vi "test_HM_times_x_preload_N22.vi"() -> ()   [LabVIEW 2017, in "MPC_FXP_FGM_TestCase.lvclass"]
uses:
  MPC_FXP_FGM_TestCase.lvclass
  fpga_VIs/fixed-point/typeDefs/x_vec_type.ctl
  C:/Program Files (x86)/National Instruments/LabVIEW 2017/vi.lib/addons/_JKI Toolkits/VI Tester/TestCase.llb/TestCase.lvclass
  <vilib>/rvi/DesktopExecutionNode/Execution/niFpgaDEN_Execute.vi
  <vilib>/rvi/DesktopExecutionNode/DesktopExecutionNode.xnode
  <userlib>/_VITAC/VITAC.lvlib
panel:
  out "error out":errorcluster
  in  "error in (no error)":errorcluster
  out "MPC_FXP_FGM_TestCase.lvclass 2":refnum<class "MPC_FXP_FGM_TestCase.lvclass">
  in  "MPC_FXP_FGM_TestCase.lvclass":refnum<class "MPC_FXP_FGM_TestCase.lvclass">
  out "all rows":dbl[][](array[numeric])
  out "x_vec":T1=[0.6000000238418579, 0.6000000238418579, -0.5999999940395355, -0.5999999940395355, 0.6000000238418579, 0.6000000238418579, 0.6000000238418579, 0.6000000238418579, -0.5999999940395355, 0.6000000238418579, -0.5999999940395355, -4.0, 0.0, 0.0, 0.0, 0.0, 0.0, 0.0, 0.0, 0.0, 0.0, 0.0, 0.0, 0.0, 0.0]
  out "A*x (expected, fxp)":fxp<+/-,32,3>[](array[numeric])
  out "Ncol":u16
  out "primary_write_addr":u16
  in  "preload_vec":fxp<+/-,32,3>[](array[numeric])=[0.0, 0.0, 0.0, 0.0, 0.0, 0.0, 0.0, 0.0, 0.0, 0.0, 0.0, 0.0, 0.0, 0.0, 0.0, 0.0, 0.0, 0.0, 0.0, 0.0, 0.0, 0.0]
  out "preload_addr":u16
  out "StartIndex":u16
  out "primary result (A*x)":fxp<+/-,32,2>[](array[numeric])
  out "preload result":fxp<+/-,32,2>[](array[numeric])
  in  "SLMAX":fxp<+/-,18,5>=10.0
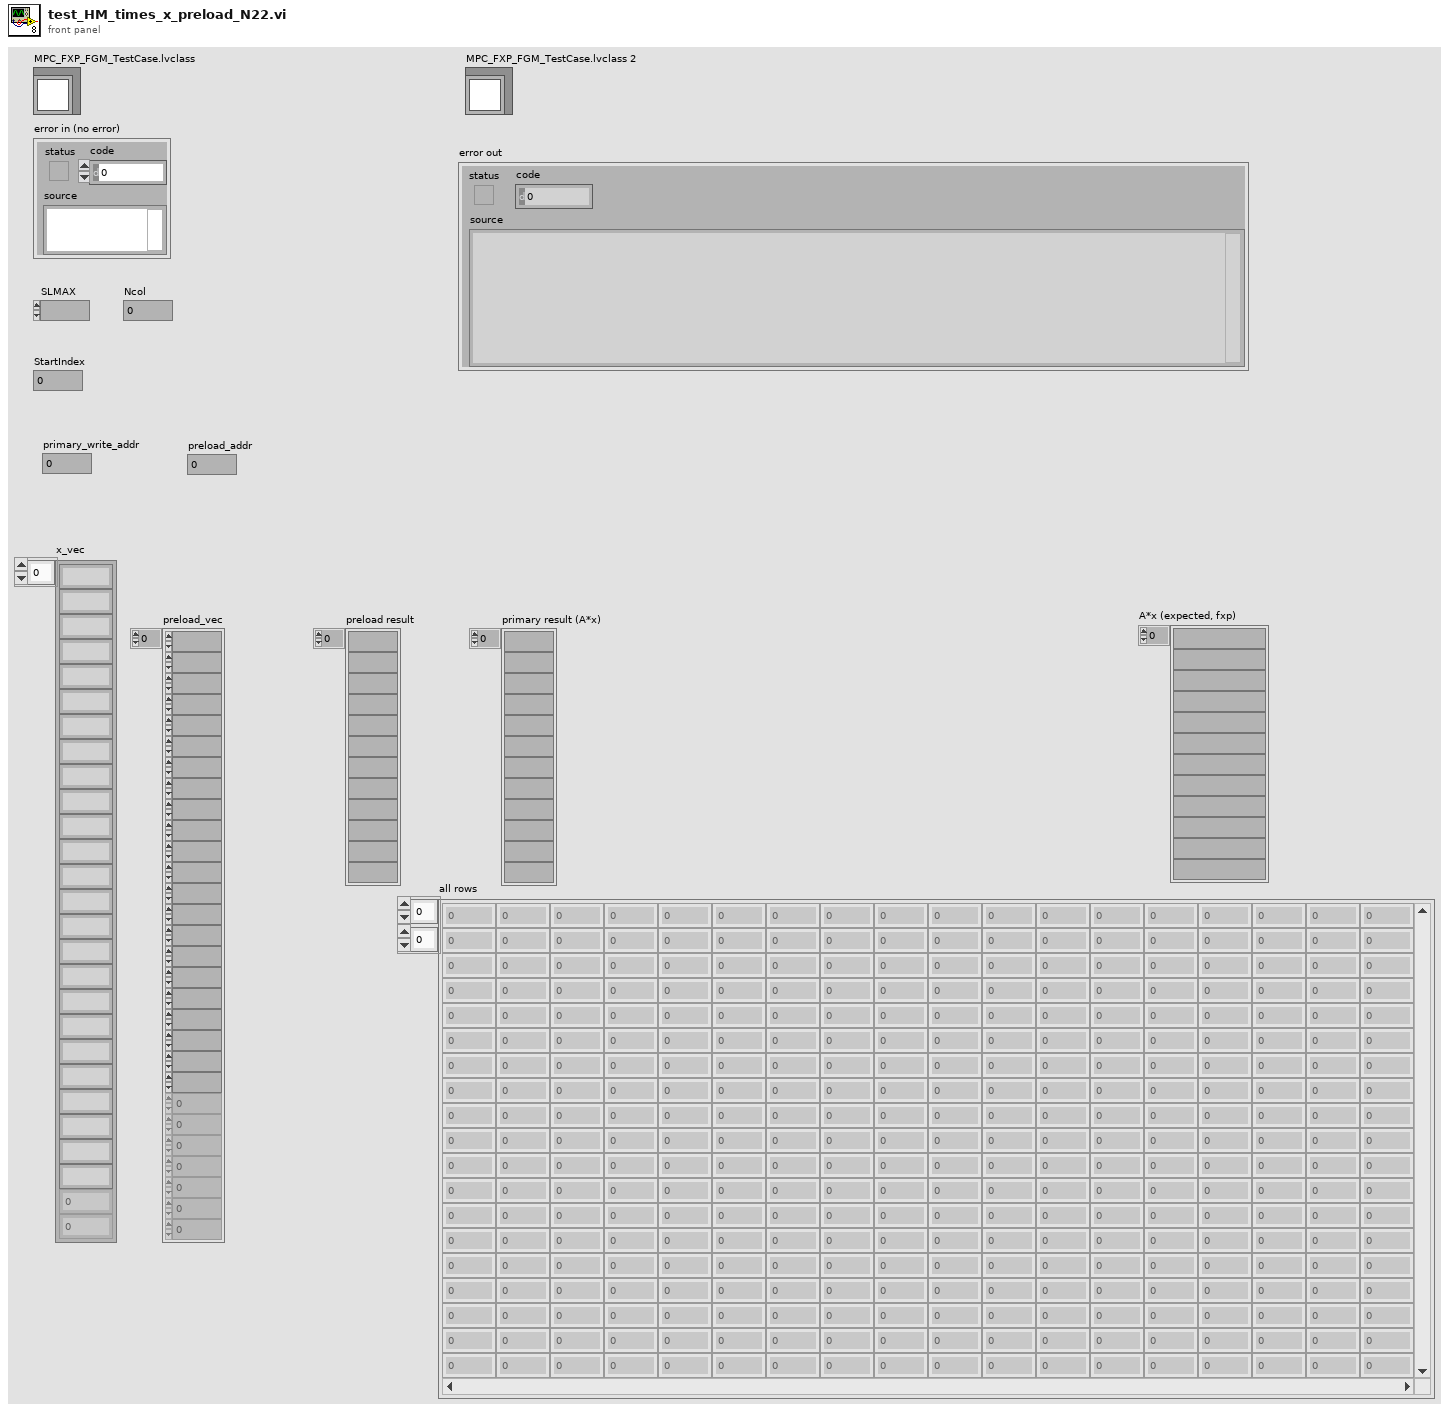
[diagram p1: front panel]
types:
  T1 = typedef "x_vec_type.ctl" = fxp<+/-,32,6>[]
  T2 = typedef "fgm_result_test_data.ctl" = cluster{"z_i_sequence":dbl[][], "y_i_sequence":dbl[][], "X_states":dbl[][]}
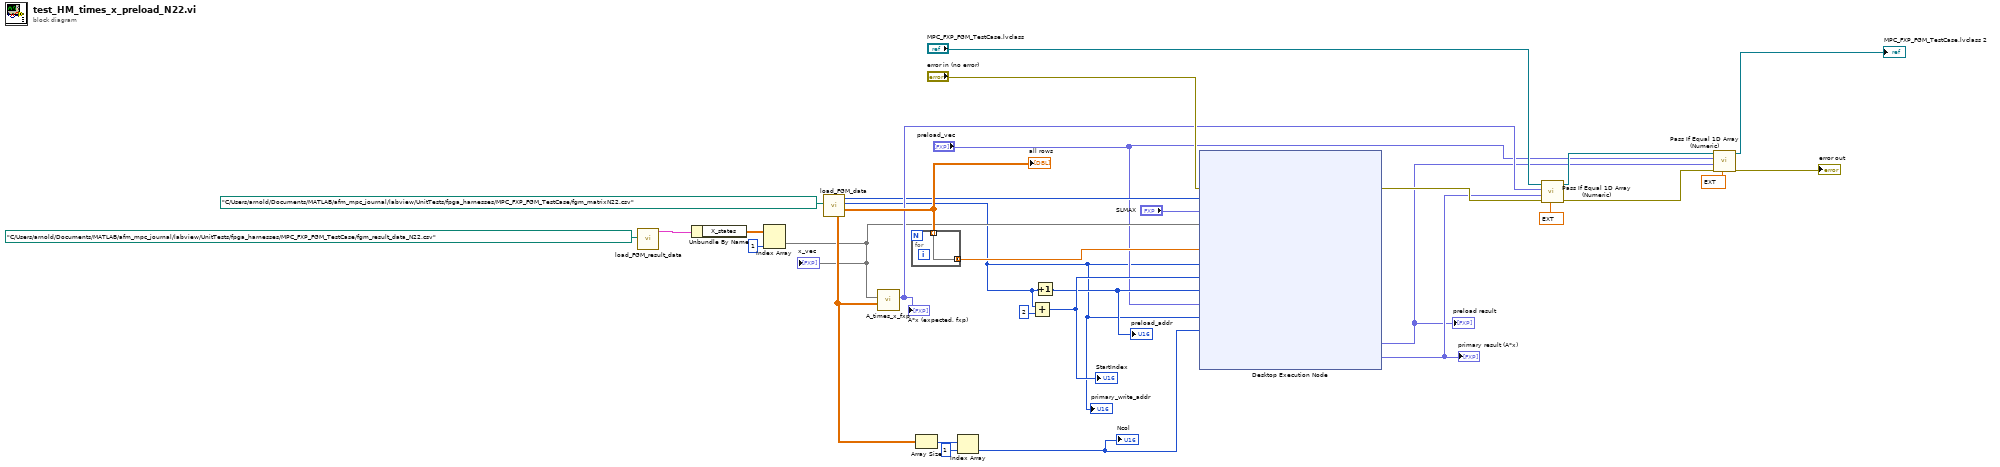
[diagram p0: block diagram]
diagram:
  n1 = call "load_FGM_result_data.vi"("Path"=path "C:/Users/arnold/Documents/MATLAB/afm_mpc_journal/labview/UnitTests/fpga_harnesses/MPC_FXP_FGM_TestCase/fgm_result_data_N22.csv") -> ("FGM_result_data"=w30:T2)  [unwired: 8 in, 2 out]
  n2 = Unbundle By Name(w30) -> ("X_states"=w29:dbl[][])
  n3 = Index Array(array=w29, index (col)=1 ("disabled index (col)")) -> (element=w11:dbl[])  [unwired: 1 in]
  "x_vec" <- w11
  n4 = call "load_FGM_data.vi"("Path"=path "C:/Users/arnold/Documents/MATLAB/afm_mpc_journal/labview/UnitTests/fpga_harnesses/MPC_FXP_FGM_TestCase/fgm_matrixN22.csv") -> ("all rows"=w31:dbl[][], "Nmpc"=w6:i32, "Ns"=w13:i32, "M"=w27:dbl[][])  [unwired: 6 in, 1 out]
  "primary_write_addr" <- w6
  "all rows" <- w31
  n5 = call "A_times_x_fxp.vi"("Az_mat in"=w27, "x_k"=w11) -> ("A*x"=w16:fxp<+/-,64,12>[])  [unwired: 8 in, 1 out]
  "A*x (expected, fxp)" <- w16
  n6 = for {
    tunnel: w31 -> [w32] mode=indexing
    tunnel: [w32] -> w10 mode=concatenating
  }
  n7 = Array Size(array=w27) -> (size(s)=w26:i32[])
  n8 = Index Array(array=w26, index=1) -> (element=w5:i32)
  "Ncol" <- w5
  n9 = Add(x=w6, y=2 ("x")) -> (x+y=w9:i32)
  "StartIndex" <- w9
  n10 = Increment(x=w6) -> (x+1=w8:i32)
  "preload_addr" <- w8
  n11 = xnode "Desktop Execution Node"("Error In"="error in (no error)", "Ns"=w13, "SLMAX"="SLMAX", "x_vec"=w11, "big_mat_data"=w10, "nuN_mpc"=w6, "StartIndex"=w9, "preload_addr"=w8, "preload_vec"="preload_vec", "primary_write_addr"=w6, "Ncol"=w5) -> ("Error Out"=w21:errorcluster, "preload result"=w3:fxp<+/-,32,3>[], "primary result"=w4:fxp<+/-,32,3>[])  [unwired: 1 out]
  "preload result" <- w3
  "primary result (A*x)" <- w4
  n12 = call <userlib>:"Pass If Equal 1D Array (Numeric).vi"("delta (optional)"=ext 0.00001, "error in (no error)"=w21, "actual"=w4, "expected"=w16, "TestCase in"="MPC_FXP_FGM_TestCase.lvclass") -> ("error out"=w20:errorcluster, "TestCase out"=w19:refnum<class "MPC_FXP_FGM_TestCase.lvclass">)  [unwired: 5 in]
  n13 = call <userlib>:"Pass If Equal 1D Array (Numeric).vi"("delta (optional)"=ext 0.00001, "error in (no error)"=w20, "actual"=w3, "expected"="preload_vec", "TestCase in"=w19) -> ("error out"=→"error out":errorcluster, "TestCase out"=→"MPC_FXP_FGM_TestCase.lvclass 2":refnum<class "MPC_FXP_FGM_TestCase.lvclass">)  [unwired: 5 in]
